vi "Get_Command_Alias.vi"(1 "Command":string, 2 "Alias Table":string[][](array[string])) -> (0 "Alias":string)   [LabVIEW 2011]
doc: "This VI finds the alias of a given \"Command\" by performing a lookup in the \"Alias Table\"."
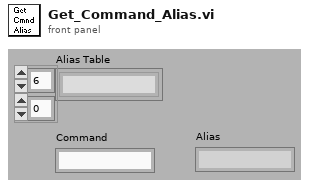
[diagram p1: front panel]
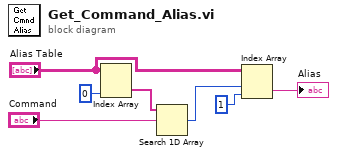
[diagram p0: block diagram]
diagram:
  n1 = Index Array(array="Alias Table", index (col)=0 ("disabled index (col)")) -> (element=w7:string[])  [unwired: 1 in]
  n2 = Search 1D Array(1D array=w7, element="Command") -> (index of element=w3:i32)  [unwired: 1 out]
  n3 = Index Array(array="Alias Table", index (row)=w3, index (col)=1 ("disabled index (col)")) -> (element=→"Alias":string)
